vi "Set CMos for CP Sweep.vi"(8 "error in (no error)":errorcluster, 11 "Control Panel":T1) -> (0 "error out":errorcluster, 1 "CP Sweep":bool, 2 "DVA":bool, 3 "E-CAL":bool)   [LabVIEW 2012]
panel:
  # "Indicator"
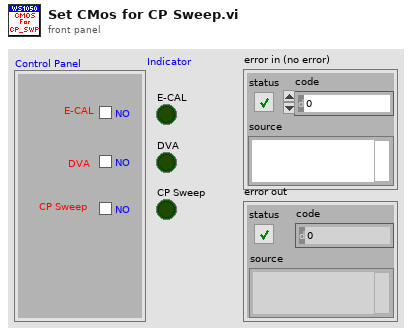
[diagram p1: front panel]
types:
  T1 = cluster{"E-CAL":bool, "DVA":bool, "CP Sweep":bool}
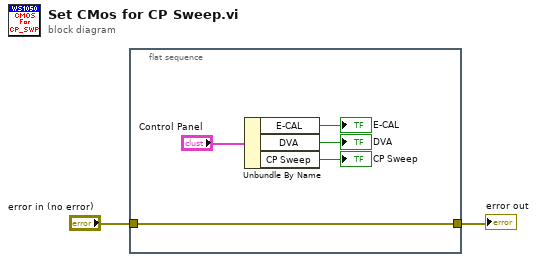
[diagram p0: block diagram]
diagram:
  n1 = flat-sequence {
    tunnel: "error in (no error)" -> [w3]
    tunnel: [w3] -> w1
    frame #0 {
      n2 = Unbundle By Name("Control Panel") -> ("E-CAL"=→"E-CAL":bool, "DVA"=→"DVA":bool, "CP Sweep"=→"CP Sweep":bool)
    }
  }
  "error out" <- w1
